vi "getScript.vi"(8 "error in (no error)":errorcluster, 11 "K2602 in":refnum<class "K2602.lvclass">) -> (0 "error out":errorcluster, 2 "script":string, 3 "K2602 out":refnum<class "K2602.lvclass">)   [LabVIEW 2011, in "Hardware.lvlib" / "Channels.lvlib" / "K2602.lvclass"]
uses:
  K2602.lvclass
  K2602.lvclass/K2602.ctl
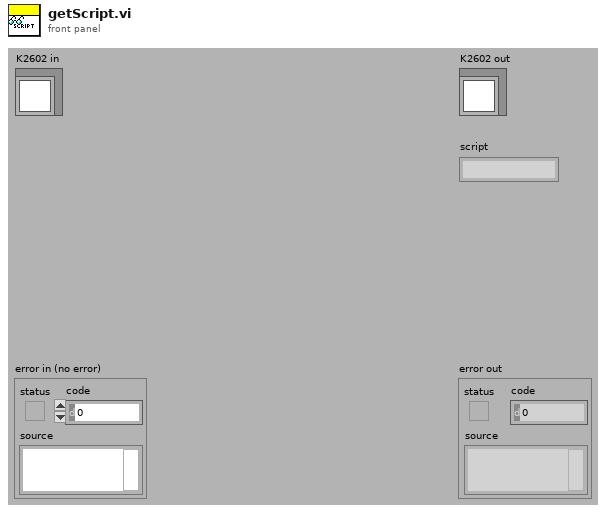
[diagram p1: front panel]
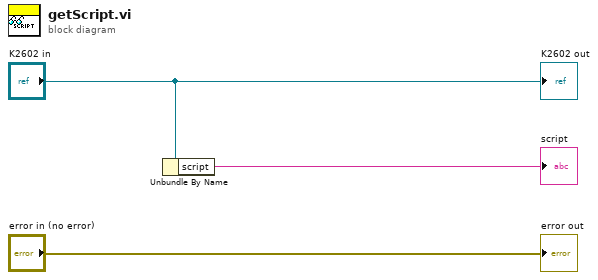
[diagram p0: block diagram]
diagram:
  n1 = Unbundle By Name("K2602 in") -> ("script"=→"script":string)
  "error out" <- "error in (no error)"
  "K2602 out" <- "K2602 in"
